vi "Emisor.vi"() -> ()   [LabVIEW 2020]
uses:
  <vilib>/Instr/_visa.llb/VISA Configure Serial Port (Instr).vi
panel:
  in  "stop":bool
  out "String":string
  out "LUZ":bool
  in  "VISA resource name":refnum<visa-resource-name>
  # "EMISOR"
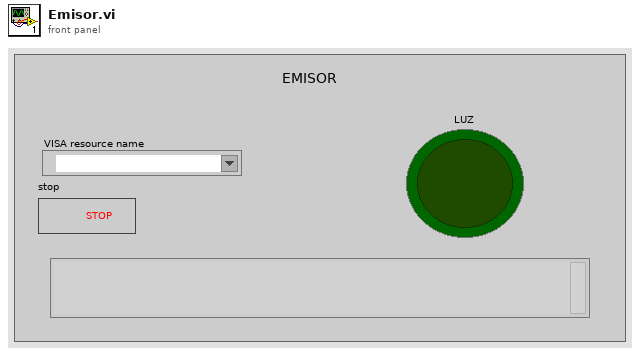
[diagram p1: front panel]
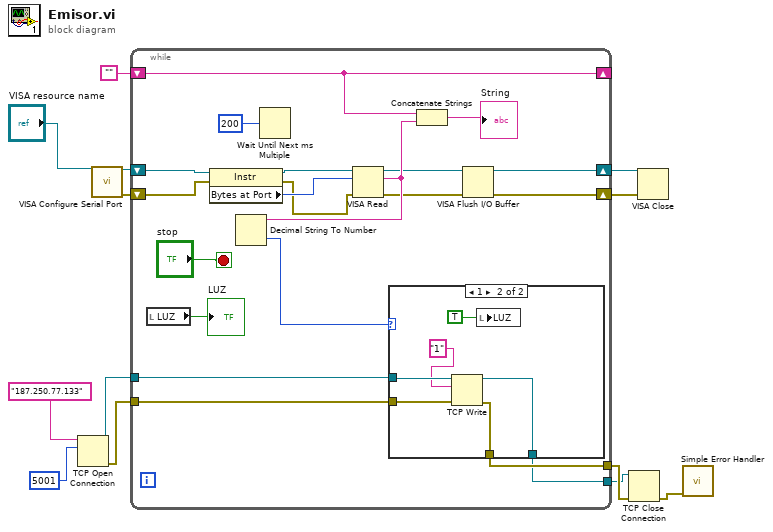
[diagram p0: block diagram]
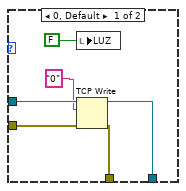
[diagram p2: hidden frame]
diagram:
  n1 = TCP Open Connection(address="187.250.77.133", remote port or service name=u16 5001) -> (connection ID=w1:refnum<k5>, error out=w2:errorcluster)  [unwired: 3 in]
  n2 = call-poly "VISA Configure Serial Port"("VISA resource name"="VISA resource name") -> ("VISA resource name out"=w13:refnum<visa-resource-name>, "error out"=w12:errorcluster)  [unwired: 13 in]
  n3 = while {
    shift-right: [w21] -> w11
    shift-left: w13 -> [w33]
    shift-right: [w19] -> w10
    shift-left: w12 -> [w32]
    shift-right: [w29] -> _
    shift-left: "" -> [w29]
    tunnel: [w17] -> w7
    tunnel: [w16] -> w6
    tunnel: w2 -> [w15]
    tunnel: w1 -> [w14]
    stop <- "stop" stop-if-true
    n4 = local read "LUZ"() -> (→"LUZ":bool)
    n5 = property class="Instr"(reference=w33, error in=w32) -> (reference out=w27:refnum<visa-resource-name>, error out=w26:errorcluster, "Bytes at Port"=w31:u32)
    n6 = Wait Until Next ms Multiple(millisecond multiple=u32 200 ("milliseconds to wait")) -> ()  [unwired: 1 out]
    n7 = VISA Read(VISA resource name=w27, byte count=w31, error in (no error)=w26) -> (VISA resource name out=w22:refnum<visa-resource-name>, read buffer=w25:string, error out=w20:errorcluster)  [unwired: 1 out]
    n8 = Decimal String To Number(string=w25) -> (number=w18:i32)  [unwired: 2 in, 1 out]
    n9 = case shown="1" w18 {
      tunnel: w15 -> [w38 w43]
      tunnel: w14 -> [w37 w44]
      tunnel: [w34 w41] -> w17
      tunnel: [w35 w40] -> w16
      frame 0, Default {
        n10 = local write "LUZ"(FALSE) -> ()
        n11 = TCP Write(connection ID=w37, data in="0", error in (no error)=w38) -> (connection ID out=w35:refnum<k5>, error out=w34:errorcluster)  [unwired: 1 in, 1 out]
      }
      frame 1 {
        n12 = TCP Write(connection ID=w44, data in="1", error in (no error)=w43) -> (connection ID out=w40:refnum<k5>, error out=w41:errorcluster)  [unwired: 1 in, 1 out]
        n13 = local write "LUZ"(TRUE) -> ()
      }
    }
    n14 = Concatenate Strings(w29, w25) -> (→"String":string)
    n15 = VISA Flush I/O Buffer(VISA resource name=w22, error in (no error)=w20) -> (VISA resource name out=w21:refnum<visa-resource-name>, error out=w19:errorcluster)  [unwired: 1 in]
  }
  n16 = TCP Close Connection(connection ID=w6, error in (no error)=w7) -> (error out=w5:errorcluster)  [unwired: 1 in, 1 out]
  n17 = VISA Close(VISA resource name=w11, error in (no error)=w10) -> ()  [unwired: 1 out]
  n18 = call <vilib>:"Simple Error Handler.vi"("error in (no error)"=w5) -> ()  [unwired: 4 in, 5 out]
